vi "meTEC_Error Test_Read_ID 100_Device Type.vi"(8 "error in (no error)":errorcluster, 9 "TEC Configuration_IN":T1={"VISA resource name"="", "Device Address"=2}, 10 "Sequence No.":u32=5552) -> (0 "error out":errorcluster, 1 "TEC Configuration_OUT":T1={"VISA resource name"="", "Device Address"=2}, 2 "Device Type (ID 100) [I32]":i32, 3 "Device Type (ID 100) [String]":string)   [LabVIEW 2019]
uses:
  TypeDefs/meTEC_Configuration.ctl
panel:
  # "--- Inputs ---"
  # "--- Outputs ---"
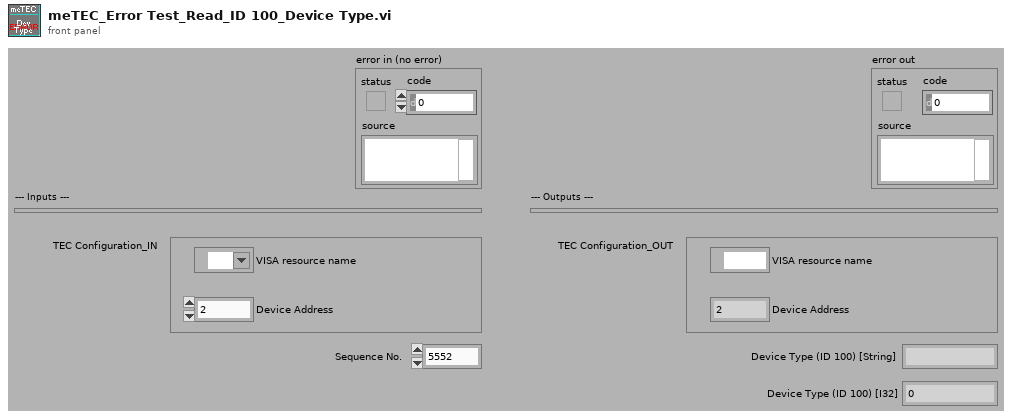
[diagram p1: front panel]
types:
  T1 = typedef "meTEC_Configuration.ctl" = cluster{"VISA resource name":refnum<visa-resource-name>, "Device Address":u16}
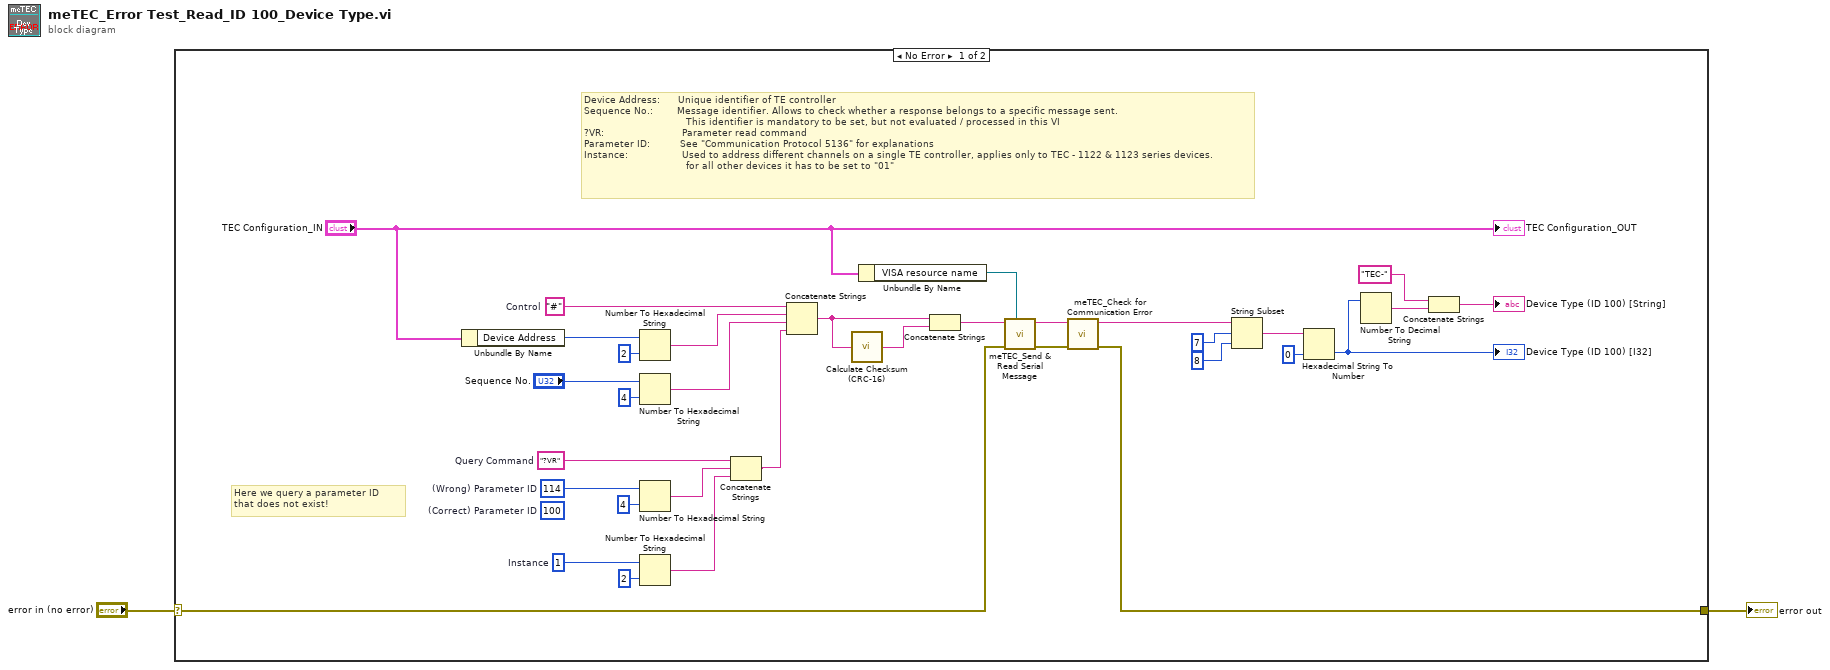
[diagram p0: block diagram]
diagram:
  n1 = case shown="No Error" "error in (no error)" {
    selector: "error in (no error)" -> [w19 w36]
    tunnel: [w5 w36] -> w2
    frame No Error {
      (unwired) 100  # (Correct) Parameter ID
      w6 = u8 1  # Instance
      w24 = 114  # (Wrong) Parameter ID
      w25 = "?VR"  # Query Command
      w33 = "#"  # Control
      # "Here we query a parameter ID\nthat does not exist!"
      # "Device Address:      Unique identifier of TE controller\nSequence No.:        Message identifier. Allows to check whether a response belongs to a specific message sent.\n                                  This identifier is mandatory to be set, but not evaluated / processed in this VI\n?VR:                          Parameter read command\nParameter ID:          See \"Communication Protocol 5136\" for explanations\nInstance:                  Used to address different channels on a single TE controller, applies only to TEC - 1122 & 1123 series devices.\n                                  for all other devices it has to be set to \"01\""
      n2 = Unbundle By Name("TEC Configuration_IN") -> ("Device Address"=w8:u16)
      n3 = Number To Hexadecimal String(1:i16 2 ("width (-)"), 2:w8) -> (0:w28:string)
      n4 = Number To Hexadecimal String(1:i16 4 ("width (-)"), 2:"Sequence No.") -> (0:w32:string)
      n5 = Number To Hexadecimal String(1:i16 4 ("width (-)"), 2:w24) -> (0:w26:string)
      n6 = Number To Hexadecimal String(1:i16 2 ("width (-)"), 2:w6) -> (0:w16:string)
      n7 = Concatenate Strings(w25, w26, w16) -> (w22:string)
      n8 = Concatenate Strings(w33, w28, w32, w22) -> (w31:string)
      n9 = call "Calculate Checksum (CRC-16).vi"("Message"=w31) -> ("CRC [String]"=w30:string)  [unwired: 1 in]
      n10 = Unbundle By Name("TEC Configuration_IN") -> ("VISA resource name"=w9:refnum<visa-resource-name>)
      n11 = Concatenate Strings(w31, w30) -> (w27:string)
      n12 = call "meTEC_Send & Read Serial Message.vi"("VISA resource name"=w9, "error in (no error)"=w19, "Serial Message"=w27) -> ("error out"=w18:errorcluster, "Serial Message_Read"=w4:string)  [unwired: 7 in]
      n13 = call "meTEC_Check for Communication Error.vi"("error in (no error)"=w18, "Serial Message_IN"=w4) -> ("error out"=w5:errorcluster, "Serial Message_OUT"=w3:string)  [unwired: 8 in]
      n14 = String Subset(string=w3, offset (0)=7, length (rest)=8 ("length (rest)")) -> (substring=w12:string)
      n15 = Hexadecimal String To Number(string=w12, default (0uL)=0 ("default (0 U32)")) -> (number=w10:i32)  [unwired: 1 in, 1 out]
      "Device Type (ID 100) [I32]" <- w10
      n16 = Number To Decimal String(number=w10) -> (decimal integer string=w11:string)  [unwired: 1 in]
      n17 = Concatenate Strings("TEC-" ("string"), w11) -> (→"Device Type (ID 100) [String]":string)
      "TEC Configuration_OUT" <- "TEC Configuration_IN"
    }
    frame Error {
    }
  }
  "error out" <- w2
